vi "4-2 AvailableDevice.vi"() -> ()   [LabVIEW 2014]
doc: "------------------------------------\nAuther: Koji Ohashi\nCopyright (c) 2020 Japan LabVIEW Users Group, Volunteer members.\nThis VI is released under the MIT License.\nhttp://opensource.org/licenses/mit-license.php\n------------------------------------"
panel:
  out "Output Device Available Parameters":T1(array[cluster])
  out "Output Device Name":string[](array[string])
  out "Input Device Available Parameters":T1(array[cluster])
  out "Input Device Name":string[](array[string])
  # "Sound Input / Output\nDevice ID, Name and Available parameters"
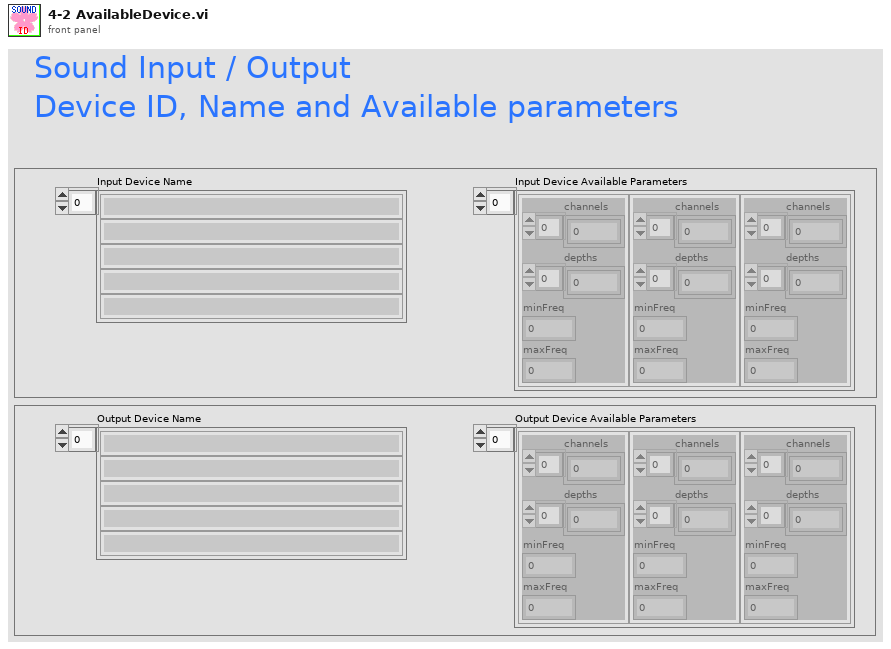
[diagram p1: front panel]
types:
  T1 = cluster{"channels":i32[], "depths":i32[], "minFreq":dbl, "maxFreq":dbl}[]
  T2 = cluster{"channels":i32[], "depths":i32[], "minFreq":dbl, "maxFreq":dbl}
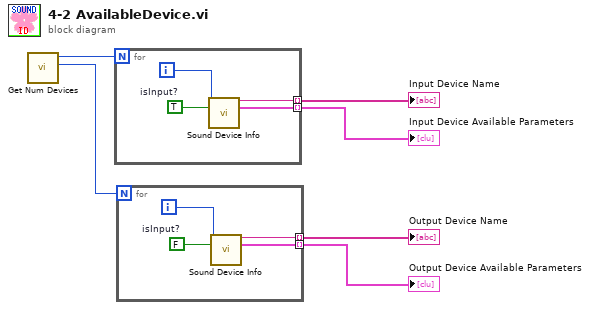
[diagram p0: block diagram]
diagram:
  n1 = call <vilib>:"Get Num Devices.vi"() -> ("Number of Output Devices"=w3:i32, "Number of Input Devices"=w6:i32)  [unwired: 9 in, 1 out]
  n2 = for {
    N: w6 -> [_]
    tunnel: [w8] -> w5 mode=indexing
    tunnel: [w7] -> w4 mode=indexing
    i -> [w9]
    w10 = TRUE  # isInput?
    n3 = call <vilib>:"Sound Device Info.vi"("device"=w9, "isInput?"=w10) -> ("Device Name"=w8:string, "Capabilities"=w7:T2)  [unwired: 11 in, 1 out]
  }
  "Input Device Name" <- w5
  "Input Device Available Parameters" <- w4
  n4 = for {
    N: w3 -> [_]
    tunnel: [w12] -> w2 mode=indexing
    tunnel: [w11] -> w1 mode=indexing
    i -> [w13]
    w14 = FALSE  # isInput?
    n5 = call <vilib>:"Sound Device Info.vi"("device"=w13, "isInput?"=w14) -> ("Device Name"=w12:string, "Capabilities"=w11:T2)  [unwired: 11 in, 1 out]
  }
  "Output Device Name" <- w2
  "Output Device Available Parameters" <- w1
